vi "Config QDFunction Shortcut In Database.vi"(8 "error in (no error)":errorcluster, 9 "QDShortcut":string, 10 "QDFullName":string, 11 "ScriptSetting in":refnum<class "ScriptSetting.lvclass">) -> (0 "error out":errorcluster, 3 "ScriptSetting out":refnum<class "ScriptSetting.lvclass">)   [LabVIEW 2015, in "ScriptSetting.lvclass"]
uses:
  ScriptSetting.lvclass
  ScriptSetting.lvclass/ScriptSetting.ctl
  _Database/Implements/ScriptDatabase.lvclass/ScriptDatabase.ctl
  QDSearchList/QDDialogList.lvclass
  _Database/Implements/ScriptDatabase.lvclass
  _Database/Ancestor/DatabaseAPI.lvclass
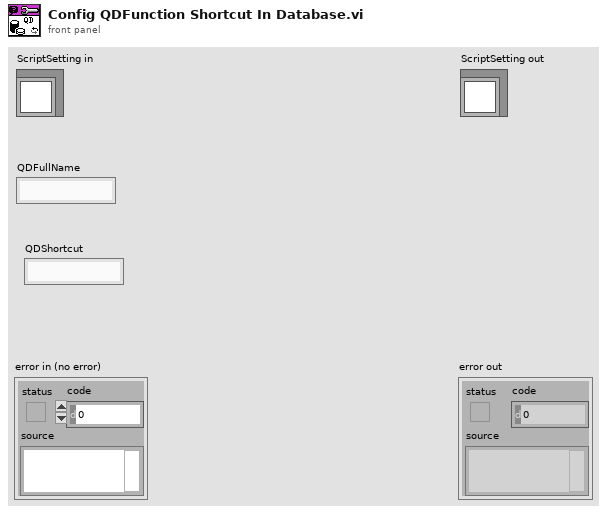
[diagram p1: front panel]
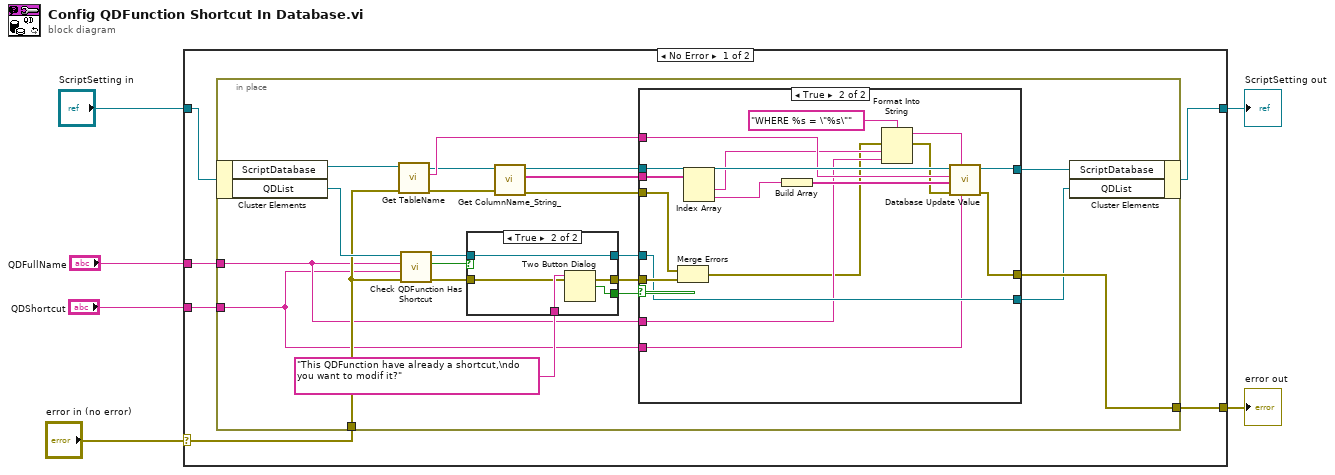
[diagram p0: block diagram]
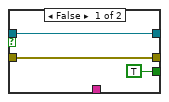
[diagram p3: hidden frame]
diagram:
  n1 = case shown="No Error" "error in (no error)" {
    selector: "error in (no error)" -> [w10 w62]
    tunnel: [w8 w62] -> w5
    tunnel: [w7 w61] -> w3
    tunnel: "ScriptSetting in" -> [w9 w61]
    tunnel: "QDFullName" -> [w12 _]
    tunnel: "QDShortcut" -> [w11 _]
    frame No Error {
      n2 = in-place {
        in-place-border: w12 -> [w20]
        in-place-border: w11 -> [w19]
        in-place-border: w10 -> [w27]
        in-place-border: [w14] -> w8
        n3 = in-place-cluster #1(w9) -> ("ScriptDatabase"=w29:refnum<class "ScriptDatabase.lvclass">, "QDList"=w30:refnum<class "QDDialogList.lvclass">)
        n4 = call "Get TableName.vi"("error in (no error)"=w27, "ScriptDatabase in"=w29) -> ("error out"=w25:errorcluster, "TableName"=w28:string, "ScriptDatabase out"=w26:refnum<class "ScriptDatabase.lvclass">)  [unwired: 7 in]
        n5 = call "Check QDFunction Has Shortcut.vi"("error in (no error)"=w27, "QDShortcut"=w19, "QDFullName"=w20, "QDDialogList in"=w30) -> ("error out"=w32:errorcluster, "HasShortcut(False)"=w33:bool, "QDDialogList out"=w22:refnum<class "QDDialogList.lvclass">)  [unwired: 5 in]
        n6 = case shown="True" w33 {
          tunnel: w32 -> [w56 w58]
          tunnel: "This QDFunction have already a shortcut,\ndo you want to modif it?" ("message") -> [_ w60]
          tunnel: [TRUE ("T button?") w59] -> w24
          tunnel: [w56 w58] -> w23
          tunnel: w22 -> [w54 w57]
          tunnel: [w54 w57] -> w21
          frame False {
          }
          frame True {
            n7 = Two Button Dialog(message=w60) -> (T button?=w59:bool)  [unwired: 2 in]
          }
        }
        n8 = call "Get ColumnName_String_.vi"("error in (no error)"=w25, "ScriptDatabase in"=w26) -> ("error out"=w17:errorcluster, "ColumnName<String>"=w16:string[], "ScriptDatabase out"=w18:refnum<class "ScriptDatabase.lvclass">)  [unwired: 7 in]
        n9 = case shown="True" w24 {
          tunnel: w28 -> [_ w44]
          tunnel: w23 -> [w34 w53]
          tunnel: w21 -> [w35 w51]
          tunnel: w20 -> [_ w40]
          tunnel: w19 -> [_ w47]
          tunnel: w18 -> [w36 w50]
          tunnel: w17 -> [_ w52]
          tunnel: w16 -> [_ w46]
          tunnel: [w34 w48] -> w14
          tunnel: [w36 w49] -> w15
          tunnel: [w35 w51] -> w13
          frame False {
          }
          frame True {
            n10 = Merge Errors(w52, w53) -> (w38:errorcluster)
            n11 = Index Array(array=w46) -> (element #1=w41:string, element #2=w42:string)  [unwired: 2 in]
            n12 = Build Array(w42) -> (w45:string[])
            n13 = Format Into String(format string="WHERE %s = \"%s\"", error in=w38, w41, w40) -> (resulting string=w39:string, error out=w37:errorcluster)  [unwired: 1 in]
            n14 = call "Database Update Value.vi"("data"=w47, "condition"=w39, "error in (no error)"=w37, "columns"=w45, "table"=w44, "Database in"=w50) -> ("error out"=w48:errorcluster, "Database out"=w49:refnum<class "ScriptDatabase.lvclass">)  [unwired: 4 in]
          }
        }
        n15 = in-place-cluster #1("ScriptDatabase"=w15, "QDList"=w13) -> (w7:refnum<class "ScriptSetting.lvclass">)
      }
    }
    frame Error {
    }
  }
  "error out" <- w5
  "ScriptSetting out" <- w3
